vi "capex data interface.vi"(2 "Save frequency":dbl=1.0, 3 "Data storage location":path=path "c:/datalogging") -> ()   [LabVIEW 2013]
panel:
  out "Output values to string":string
  out "new header":string
  out "old header":string
  out "notes refnum":refnum<file>
  out "datalogging refnum":refnum<file>
  in  "Enum":T1(ring)=enum."Initialization"
  out "Julian day":i32=237
  in  "stop":bool
  out "Low disk space":bool
  in  "Log note":bool
  in  "Notes":string
  out "Free GB":dbl
  # "seconds between saves"
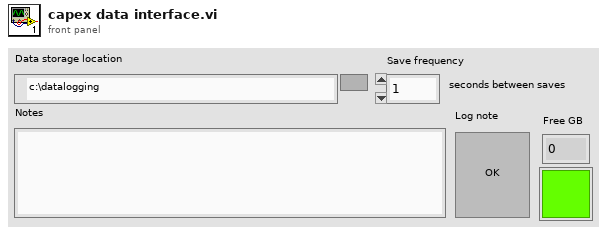
[diagram p1: front panel]
types:
  T1 = enum16{"Write all values", "Exit", "Initialization", "Logging"}
  T2 = enum16{"open", "replace", "create", "open or create", "replace or create", "replace or create with confirmation"}
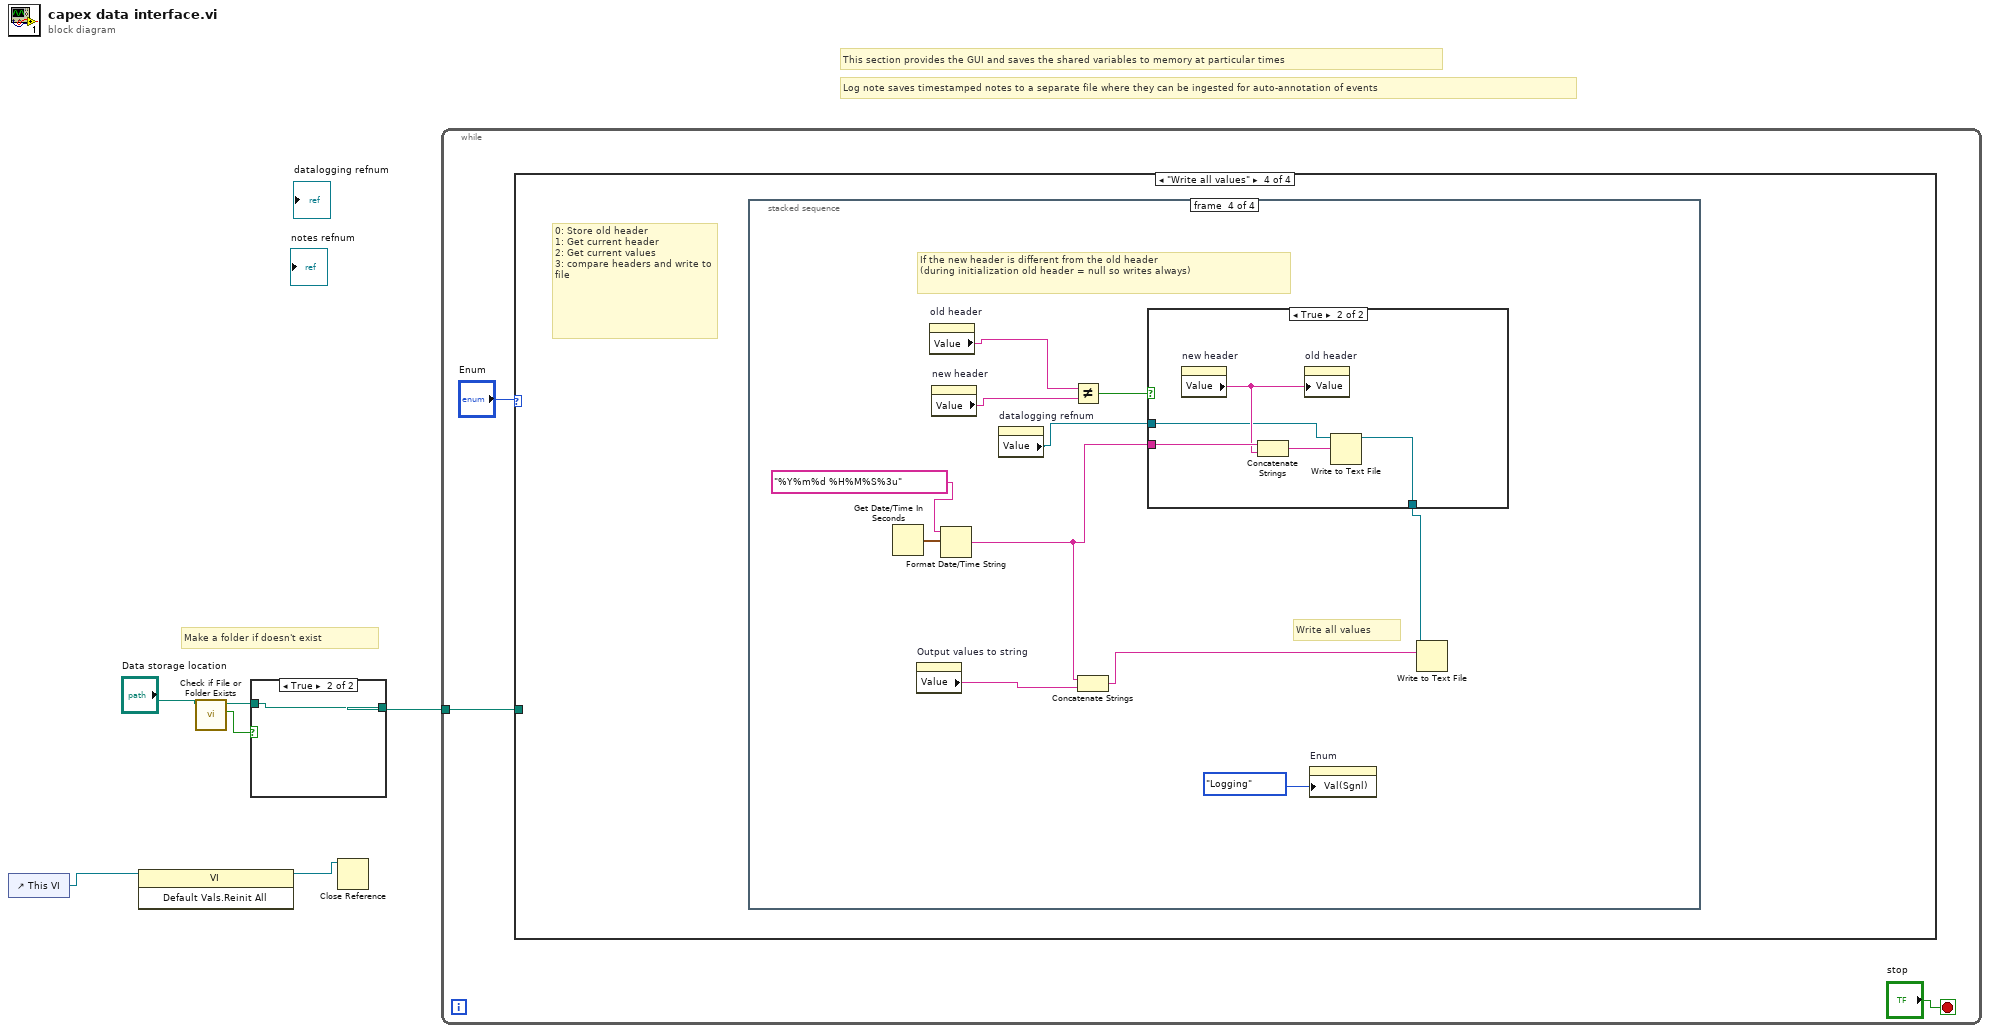
[diagram p0: block diagram]
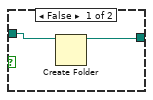
[diagram p2: hidden frame]
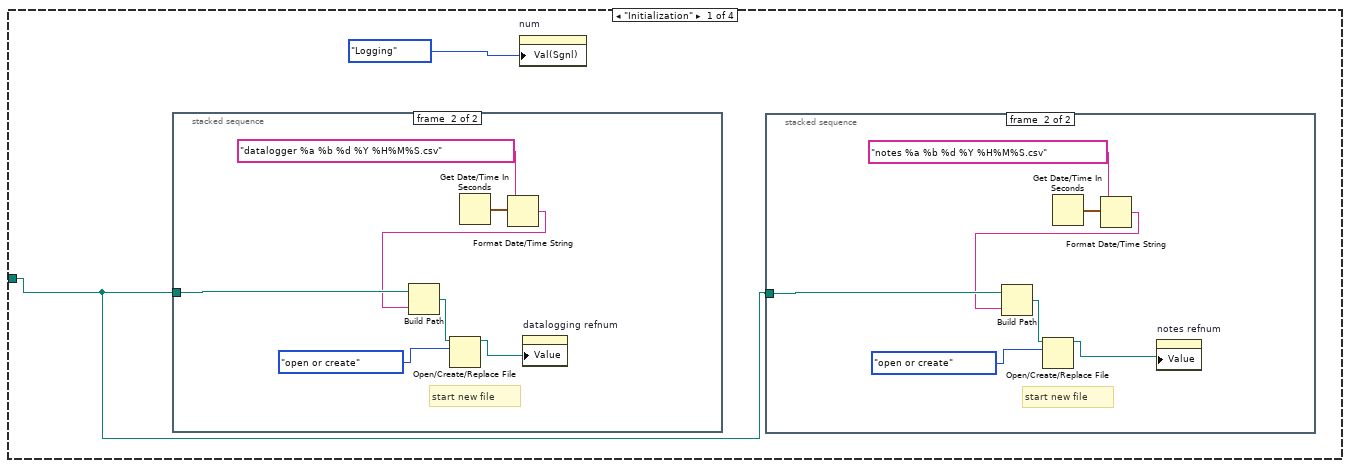
[diagram p3: hidden frame]
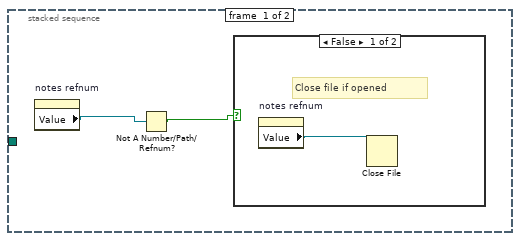
[diagram p4: hidden frame]
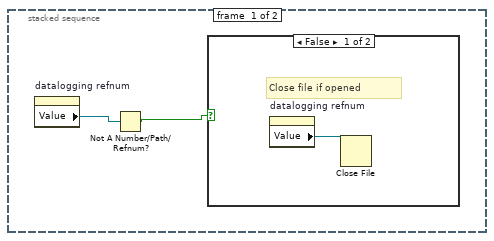
[diagram p6: hidden frame]
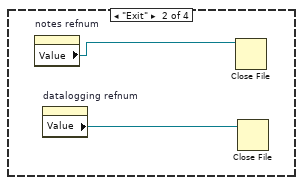
[diagram p8: hidden frame]
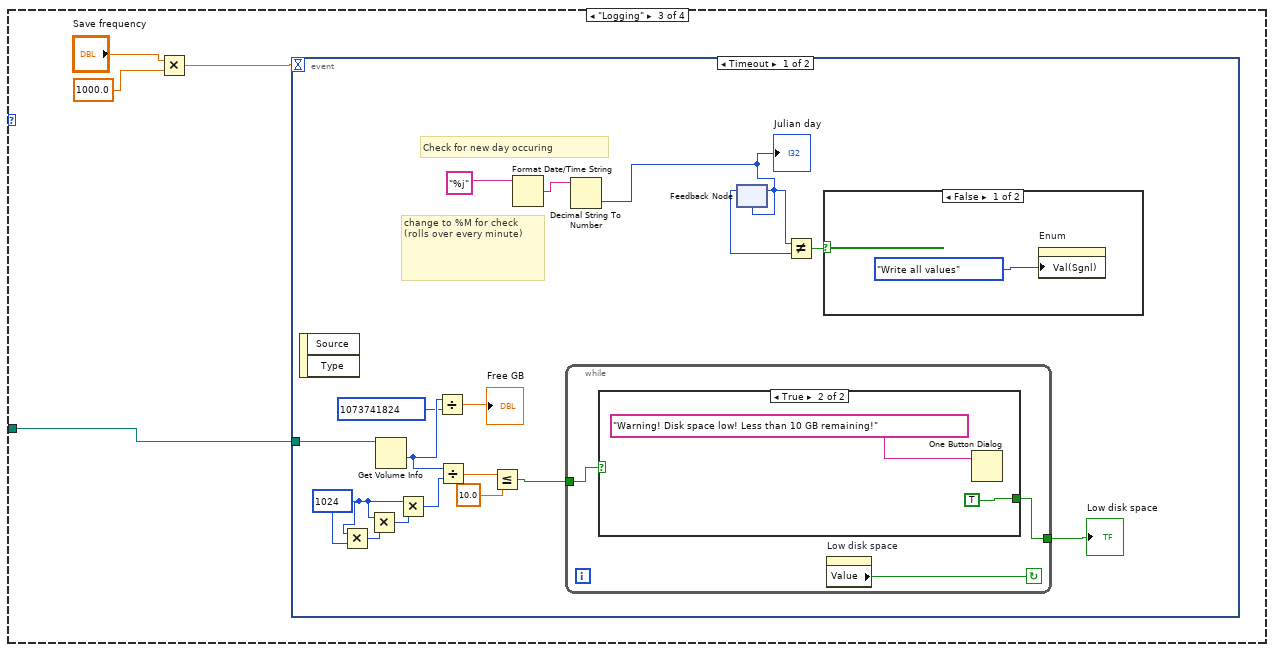
[diagram p9: hidden frame]
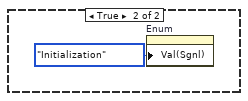
[diagram p10: hidden frame]
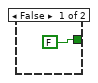
[diagram p11: hidden frame]
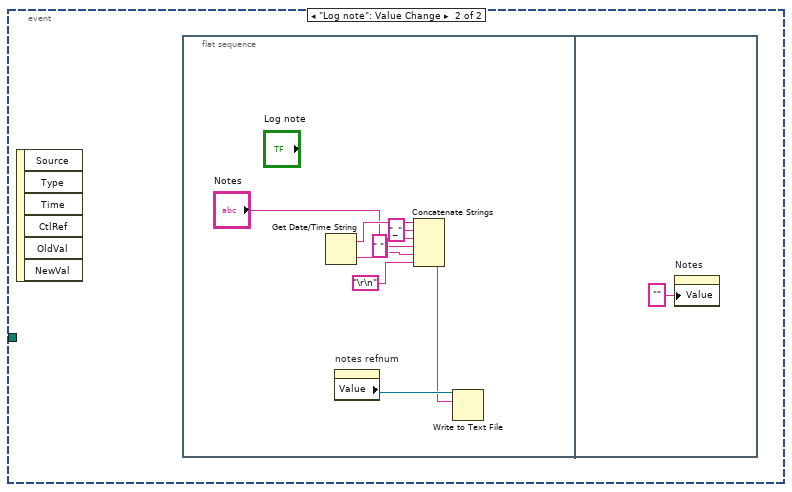
[diagram p12: hidden frame]
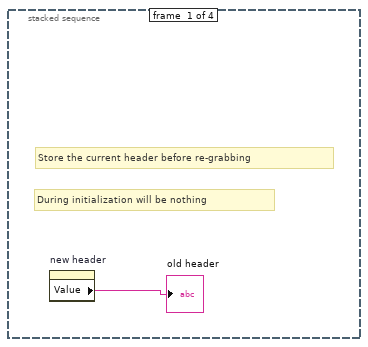
[diagram p13: hidden frame]
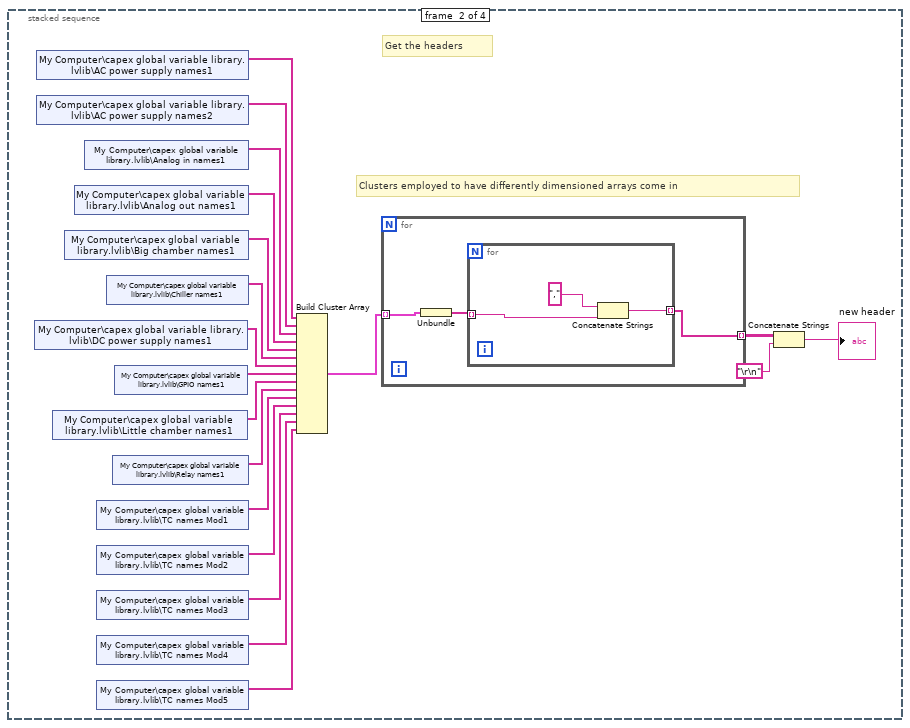
[diagram p14: hidden frame]
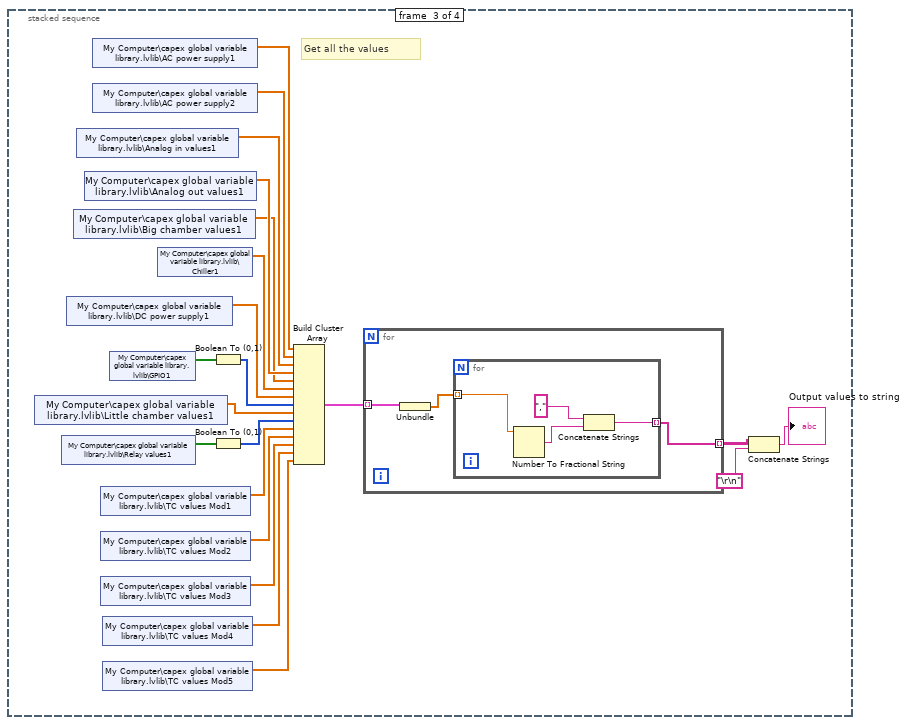
[diagram p15: hidden frame]
diagram:
  # "Make a folder if doesn't exist"
  # "Log note saves timestamped notes to a separate file where they can be ingested for auto-annotation of events"
  # "This section provides the GUI and saves the shared variables to memory at particular times"
  n1 = control-ref of="This VI"() -> (w2:refnum<vi>)
  n2 = invoke class="VI" method="Default Vals.Reinit All"(reference=w2) -> (reference out=w1:refnum<vi>)  [unwired: 2 in, 2 out]
  n3 = call <vilib>:"Check if File or Folder Exists.vi"("path"="Data storage location") -> ("file or folder exists?"=w5:bool, "dup path"=w3:path)  [unwired: 8 in, 1 out]
  n4 = case shown="True" w5 {
    tunnel: [w8 w9] -> w6
    tunnel: w3 -> [w7 w9]
    frame False {
      n5 = Create Folder(path (use dialog)=w7) -> (created path=w8:path)  [unwired: 2 in, 2 out]
    }
    frame True {
    }
  }
  n6 = Close Reference(reference=w1) -> ()  [unwired: 1 in, 1 out]
  n7 = while {
    tunnel: w6 -> [w11]
    stop <- "stop" stop-if-true
    n8 = case shown="\"Write all values\"" "Enum" {
      tunnel: w11 -> [w13 _ w37 _]
      frame "Initialization" {
        n9 = stacked-sequence {
          tunnel: w13 -> [_ w33]
          frame #0 {
            n10 = property on="datalogging refnum" class="Ref (strict)"() -> ("Value"=w25:refnum<file>)  [unwired: 2 in, 2 out]
            n11 = Not A Number/Path/Refnum?(number/path/refnum=w25) -> (NaN/Path/Refnum?=w26:bool)
            n12 = case shown="False" w26 {
              frame False {
                # "Close file if opened"
                n13 = property on="datalogging refnum" class="Ref (strict)"() -> ("Value"=w27:refnum<file>)  [unwired: 2 in, 2 out]
                n14 = Close File(refnum=w27) -> ()  [unwired: 1 in, 2 out]
              }
              frame True {
              }
            }
          }
          frame #1 {
            # "start new file"
            n15 = Get Date/Time In Seconds() -> (seconds since 1Jan1904=w30:timestamp)
            n16 = Format Date/Time String(time format string (%c)="datalogger %a %b %d %Y %H%M%S.csv", seconds (now)=w30) -> (date/time string=w28:string)  [unwired: 1 in]
            n17 = Build Path(base path=w33, name or relative path=w28) -> (appended path=w32:path)
            n18 = Open/Create/Replace File(file path (use dialog)=w32, operation (0:open)=T2."open or create") -> (refnum out=w31:refnum<file>)  [unwired: 4 in, 2 out]
            n19 = property on="datalogging refnum" class="Ref (strict)"("Value"=w31) -> ()  [unwired: 2 in, 2 out]
          }
        }
        n20 = property on="num" class="Enum (strict)"("Val(Sgnl)"=T1."Logging" ("Value (Signaling)")) -> ()  [unwired: 2 in, 2 out]
        n21 = stacked-sequence {
          tunnel: w13 -> [_ w23]
          frame #0 {
            n22 = property on="notes refnum" class="Ref (strict)"() -> ("Value"=w15:refnum<file>)  [unwired: 2 in, 2 out]
            n23 = Not A Number/Path/Refnum?(number/path/refnum=w15) -> (NaN/Path/Refnum?=w16:bool)
            n24 = case shown="False" w16 {
              frame False {
                # "Close file if opened"
                n25 = property on="notes refnum" class="Ref (strict)"() -> ("Value"=w17:refnum<file>)  [unwired: 2 in, 2 out]
                n26 = Close File(refnum=w17) -> ()  [unwired: 1 in, 2 out]
              }
              frame True {
              }
            }
          }
          frame #1 {
            # "start new file"
            n27 = Get Date/Time In Seconds() -> (seconds since 1Jan1904=w21:timestamp)
            n28 = Format Date/Time String(time format string (%c)="notes %a %b %d %Y %H%M%S.csv", seconds (now)=w21) -> (date/time string=w19:string)  [unwired: 1 in]
            n29 = Build Path(base path=w23, name or relative path=w19) -> (appended path=w22:path)
            n30 = Open/Create/Replace File(file path (use dialog)=w22, operation (0:open)=T2."open or create") -> (refnum out=w18:refnum<file>)  [unwired: 4 in, 2 out]
            n31 = property on="notes refnum" class="Ref (strict)"("Value"=w18) -> ()  [unwired: 2 in, 2 out]
          }
        }
      }
      frame "Exit" {
        n32 = property on="notes refnum" class="Ref (strict)"() -> ("Value"=w36:refnum<file>)  [unwired: 2 in, 2 out]
        n33 = property on="datalogging refnum" class="Ref (strict)"() -> ("Value"=w35:refnum<file>)  [unwired: 2 in, 2 out]
        n34 = Close File(refnum=w36) -> ()  [unwired: 1 in, 2 out]
        n35 = Close File(refnum=w35) -> ()  [unwired: 1 in, 2 out]
      }
      frame "Logging" {
        n36 = Multiply(x="Save frequency", y=1000.0) -> (x*y=w38:dbl)
        n37 = event shown="[0] Timeout" {
          selector: _ -> [_ _]
          dyn-events: _ -> [_ _]
          timeout: w38 -> [_ _]
          tunnel: w37 -> [w53 _]
          event Timeout {
            w54 = 1024
            # "change to %M for check (rolls over every minute)"
            # "Check for new day occuring"
            n38 = event-data() -> ()  [unwired: 1 in, 2 out]
            n39 = Multiply(x=w54, y=w54) -> (x*y=w57:i32)
            n40 = Multiply(x=w54, y=w57) -> (x*y=w56:i32)
            n41 = Get Volume Info(11:w53) -> (1:w43:i64)  [unwired: 1 in, 5 out]
            n42 = Multiply(x=w54, y=w56) -> (x*y=w55:i32)
            n43 = Divide(x=w43, y=i64 1073741824) -> (x/y=→"Free GB":dbl)
            n44 = Divide(x=w43, y=w55) -> (x/y=w52:dbl)
            n45 = Less Or Equal?(x=w52, y=10.0) -> (x <= y?=w49:bool)
            n46 = Format Date/Time String(time format string (%c)="%j") -> (date/time string=w46:string)  [unwired: 2 in]
            n47 = while {
              tunnel: [w62] -> w50
              tunnel: w49 -> [w61]
              stop <- w60 continue-if-true
              n48 = case shown="True" w61 {
                tunnel: [FALSE TRUE] -> w62
                frame False {
                }
                frame True {
                  n49 = One Button Dialog(message="Warning! Disk space low! Less than 10 GB remaining!") -> ()  [unwired: 1 in, 1 out]
                }
              }
              n50 = property on="Low disk space" class="Bool (strict)"() -> ("Value"=w60:bool)  [unwired: 2 in, 2 out]
            }
            "Low disk space" <- w50
            n51 = Decimal String To Number(string=w46) -> (number=w45:i32)  [unwired: 2 in, 1 out]
            "Julian day" <- w45
            n52 = feedback #1(w45) -> (w48:i32)
            n53 = feedback-in #1(w45) -> ()
            n54 = Not Equal?(x=w45, y=w48) -> (x != y?=w44:bool)
            n55 = case shown="False" w44 {
              frame False {
                n56 = property on="Enum" class="Enum (strict)"("Val(Sgnl)"=T1."Write all values" ("Value (Signaling)")) -> ()  [unwired: 2 in, 2 out]
              }
              frame True {
                n57 = property on="Enum" class="Enum (strict)"("Val(Sgnl)"=T1."Initialization" ("Value (Signaling)")) -> ()  [unwired: 2 in, 2 out]
              }
            }
          }
          event "Log note": Value Change {
            n58 = event-data() -> ()  [unwired: 1 in, 6 out]
            n59 = flat-sequence {
              frame #0 {
                n60 = Get Date/Time String() -> (date string=w72:string, time string=w71:string)  [unwired: 3 in]
                n61 = property on="notes refnum" class="Ref (strict)"() -> ("Value"=w73:refnum<file>)  [unwired: 2 in, 2 out]
                n62 = Concatenate Strings(w72, "_" ("element"), w71, " " ("string"), "Notes", "\r\n") -> (w69:string)
                n63 = Write to Text File(file (use dialog)=w73, text=w69) -> ()  [unwired: 2 in, 3 out]
              }
              frame #1 {
                n64 = property on="Notes" class="Str"("Value"="" ("Notes")) -> ()  [unwired: 2 in, 2 out]
              }
            }
          }
        }
      }
      frame "Write all values" {
        # "0: Store old header\n1: Get current header\n2: Get current values\n3: compare headers and write to file"
        n65 = stacked-sequence {
          frame #0 {
            # "During initialization will be nothing"
            # "Store the current header before re-grabbing"
            n66 = property on="new header" class="Str"() -> ("Value"=→"old header":string)  [unwired: 2 in, 2 out]
          }
          frame #1 {
            # "Clusters employed to have differently dimensioned arrays come in"
            # "Get the headers"
            n67 = shared-variable "My Computer\\capex global variable library.lvlib\\DC power supply names1"() -> (w85:string[])  [unwired: 1 in, 1 out]
            n68 = shared-variable "My Computer\\capex global variable library.lvlib\\AC power supply names1"() -> (w76:string[])  [unwired: 1 in, 1 out]
            n69 = shared-variable "My Computer\\capex global variable library.lvlib\\AC power supply names2"() -> (w90:string[])  [unwired: 1 in, 1 out]
            n70 = shared-variable "My Computer\\capex global variable library.lvlib\\Little chamber names1"() -> (w83:string[])  [unwired: 1 in, 1 out]
            n71 = shared-variable "My Computer\\capex global variable library.lvlib\\Big chamber names1"() -> (w87:string[])  [unwired: 1 in, 1 out]
            n72 = shared-variable "My Computer\\capex global variable library.lvlib\\Analog out names1"() -> (w88:string[])  [unwired: 1 in, 1 out]
            n73 = shared-variable "My Computer\\capex global variable library.lvlib\\Analog in names1"() -> (w89:string[])  [unwired: 1 in, 1 out]
            n74 = shared-variable "My Computer\\capex global variable library.lvlib\\TC names Mod1"() -> (w81:string[])  [unwired: 1 in, 1 out]
            n75 = shared-variable "My Computer\\capex global variable library.lvlib\\TC names Mod2"() -> (w80:string[])  [unwired: 1 in, 1 out]
            n76 = shared-variable "My Computer\\capex global variable library.lvlib\\TC names Mod3"() -> (w79:string[])  [unwired: 1 in, 1 out]
            n77 = shared-variable "My Computer\\capex global variable library.lvlib\\TC names Mod4"() -> (w78:string[])  [unwired: 1 in, 1 out]
            n78 = shared-variable "My Computer\\capex global variable library.lvlib\\TC names Mod5"() -> (w77:string[])  [unwired: 1 in, 1 out]
            n79 = shared-variable "My Computer\\capex global variable library.lvlib\\Chiller names1"() -> (w86:string[])  [unwired: 1 in, 1 out]
            n80 = shared-variable "My Computer\\capex global variable library.lvlib\\Relay names1"() -> (w82:string[])  [unwired: 1 in, 1 out]
            n81 = shared-variable "My Computer\\capex global variable library.lvlib\\GPIO names1"() -> (w84:string[])  [unwired: 1 in, 1 out]
            n82 = Build Cluster Array(w76, w90, w89, w88, w87, w86, w85, w84, w83, w82, w81, w80, w79, w78, w77) -> (w94:cluster{"Array of String":string[]}[])
            n83 = for {
              tunnel: w94 -> [w96] mode=indexing
              tunnel: [w97] -> w93 mode=indexing
              n84 = Unbundle(w96) -> ("Array of String"=w95:string[])
              n85 = for {
                tunnel: [w99] -> w97 mode=indexing
                tunnel: w95 -> [w98] mode=indexing
                n86 = Concatenate Strings("," ("string"), w98) -> (w99:string)
              }
            }
            n87 = Concatenate Strings(w93, "\r\n") -> (→"new header":string)
          }
          frame #2 {
            # "Get all the values"
            n88 = shared-variable "My Computer\\capex global variable library.lvlib\\Little chamber values1"() -> (w115:dbl[])  [unwired: 1 in, 1 out]
            n89 = shared-variable "My Computer\\capex global variable library.lvlib\\Relay values1"() -> (w120:bool[])  [unwired: 1 in, 1 out]
            n90 = shared-variable "My Computer\\capex global variable library.lvlib\\DC power supply1"() -> (w103:dbl[])  [unwired: 1 in, 1 out]
            n91 = shared-variable "My Computer\\capex global variable library.lvlib\\Big chamber values1"() -> (w104:dbl[])  [unwired: 1 in, 1 out]
            n92 = shared-variable "My Computer\\capex global variable library.lvlib\\Analog in values1"() -> (w118:dbl[])  [unwired: 1 in, 1 out]
            n93 = shared-variable "My Computer\\capex global variable library.lvlib\\Analog out values1"() -> (w105:dbl[])  [unwired: 1 in, 1 out]
            n94 = shared-variable "My Computer\\capex global variable library.lvlib\\AC power supply1"() -> (w119:dbl[])  [unwired: 1 in, 1 out]
            n95 = shared-variable "My Computer\\capex global variable library.lvlib\\AC power supply2"() -> (w102:dbl[])  [unwired: 1 in, 1 out]
            n96 = shared-variable "My Computer\\capex global variable library.lvlib\\TC values Mod1"() -> (w113:dbl[])  [unwired: 1 in, 1 out]
            n97 = shared-variable "My Computer\\capex global variable library.lvlib\\TC values Mod2"() -> (w112:dbl[])  [unwired: 1 in, 1 out]
            n98 = shared-variable "My Computer\\capex global variable library.lvlib\\TC values Mod3"() -> (w111:dbl[])  [unwired: 1 in, 1 out]
            n99 = shared-variable "My Computer\\capex global variable library.lvlib\\TC values Mod4"() -> (w110:dbl[])  [unwired: 1 in, 1 out]
            n100 = shared-variable "My Computer\\capex global variable library.lvlib\\TC values Mod5"() -> (w101:dbl[])  [unwired: 1 in, 1 out]
            n101 = shared-variable "My Computer\\capex global variable library.lvlib\\GPIO1"() -> (w121:bool[])  [unwired: 1 in, 1 out]
            n102 = shared-variable "My Computer\\capex global variable library.lvlib\\Chiller1"() -> (w117:dbl[])  [unwired: 1 in, 1 out]
            n103 = Boolean To (0,1)(Boolean=w121) -> (0, 1=w116:i16[])
            n104 = Boolean To (0,1)(Boolean=w120) -> (0, 1=w114:i16[])
            n105 = Build Cluster Array(w119, w102, w118, w105, w104, w117, w103, w116, w115, w114, w113, w112, w111, w110, w101) -> (w109:cluster{"Array of Double":dbl[]}[])
            n106 = for {
              tunnel: w109 -> [w123] mode=indexing
              tunnel: [w124] -> w107 mode=indexing
              n107 = Unbundle(w123) -> ("Array of Double"=w122:dbl[])
              n108 = for {
                tunnel: w122 -> [w125] mode=indexing
                tunnel: [w127] -> w124 mode=indexing
                n109 = Number To Fractional String(number=w125) -> (F-format string=w126:string)  [unwired: 3 in]
                n110 = Concatenate Strings("," ("string"), w126) -> (w127:string)
              }
            }
            n111 = Concatenate Strings(w107, "\r\n") -> (→"Output values to string":string)
          }
          frame #3 {
            # "Write all values"
            # "If the new header is different from the old header\n(during initialization old header = null so writes always)"
            n112 = Get Date/Time In Seconds() -> (seconds since 1Jan1904=w136:timestamp)
            n113 = property on="Output values to string" class="Str"() -> ("Value"=w133:string)  [unwired: 2 in, 2 out]
            n114 = property on="old header" class="Str"() -> ("Value"=w139:string)  [unwired: 2 in, 2 out]
            n115 = property on="new header" class="Str"() -> ("Value"=w138:string)  [unwired: 2 in, 2 out]
            n116 = Format Date/Time String(time format string (%c)="%Y%m%d %H%M%S%3u", seconds (now)=w136) -> (date/time string=w134:string)  [unwired: 1 in]
            n117 = property on="datalogging refnum" class="Ref (strict)"() -> ("Value"=w132:refnum<file>)  [unwired: 2 in, 2 out]
            n118 = Not Equal?(x=w139, y=w138) -> (x != y?=w137:bool)
            n119 = Concatenate Strings(w134, w133) -> (w129:string)
            n120 = case shown="True" w137 {
              tunnel: w134 -> [_ w145]
              tunnel: w132 -> [w140 w143]
              tunnel: [w140 w142] -> w131
              frame False {
              }
              frame True {
                n121 = property on="new header" class="Str"() -> ("Value"=w144:string)  [unwired: 2 in, 2 out]
                n122 = Concatenate Strings(w145, w144) -> (w141:string)
                n123 = property on="old header" class="Str"("Value"=w144) -> ()  [unwired: 2 in, 2 out]
                n124 = Write to Text File(file (use dialog)=w143, text=w141) -> (refnum out=w142:refnum<file>)  [unwired: 2 in, 2 out]
              }
            }
            n125 = property on="Enum" class="Enum (strict)"("Val(Sgnl)"=T1."Logging" ("Value (Signaling)")) -> ()  [unwired: 2 in, 2 out]
            n126 = Write to Text File(file (use dialog)=w131, text=w129) -> ()  [unwired: 2 in, 3 out]
          }
        }
      }
    }
  }
